vi "SRV_Update Main Window Title and Open Window.vi"(0 "VI ref":refnum<vi>, 11 "error in (no error)":errorcluster, 12 "FP.Open? (T)":bool=TRUE) -> (4 "VI ref out":refnum<vi>, 15 "error out":errorcluster)   [LabVIEW 2009]
doc: "Updates the FrontPanel.Title property of the referenced VI. The title will be \"SRV Main Controller\" plus a version number if one exists at the end of the VI filename.\n\n\nAuthor: Mike Schultz - Logic PD"
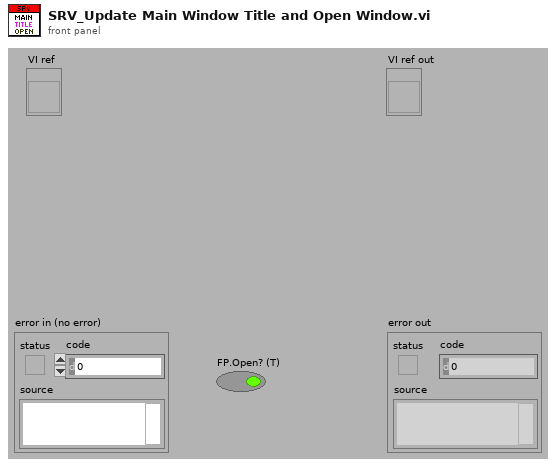
[diagram p1: front panel]
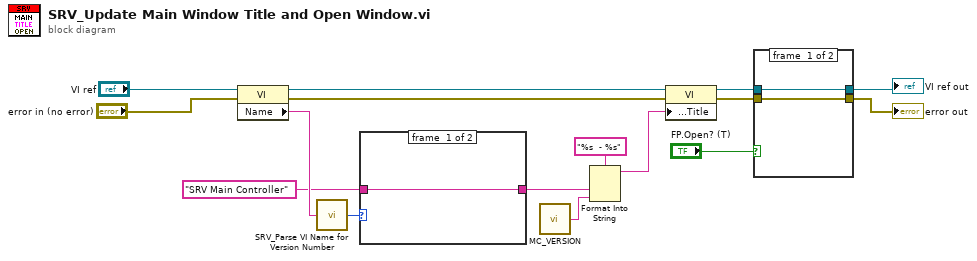
[diagram p0: block diagram]
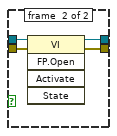
[diagram p2: hidden frame]
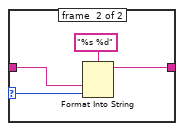
[diagram p3: hidden frame]
diagram:
  n1 = property class="VI"(reference="VI ref", error in="error in (no error)") -> (reference out=w12:refnum<vi>, error out=w11:errorcluster, "Name"=w15:string)
  n2 = call "SRV_Parse VI Name for Version Number.vi"("VI Name"=w15) -> ("Version Number"=w14:i32)  [unwired: 14 in]
  n3 = case shown="Default" w14 {
    selector: w14 -> [_ w18]
    tunnel: "SRV Main Controller" -> [w17 w20]
    tunnel: [w17 w19] -> w4
    frame #0 {
    }
    frame #1 {
      n4 = Format Into String(format string="%s %d", w20, w18) -> (resulting string=w19:string)  [unwired: 2 in, 1 out]
    }
  }
  n5 = call "MC_VERSION.vi"() -> ("MC Version"=w2:string)
  n6 = Format Into String(format string="%s  - %s", w4, w2) -> (resulting string=w3:string)  [unwired: 2 in, 1 out]
  n7 = property class="VI"(reference=w12, error in=w11, "Front Panel.Title"=w3) -> (reference out=w7:refnum<vi>, error out=w9:errorcluster)
  n8 = case shown="True" "FP.Open? (T)" {
    tunnel: w9 -> [w23 w27]
    tunnel: [w23 w26] -> w8
    tunnel: w7 -> [w22 w25]
    tunnel: [w22 w24] -> w6
    frame #0 {
    }
    frame #1 {
      n9 = invoke class="VI" method="FP.Open"(reference=w25, error in=w27) -> (reference out=w24:refnum<vi>, error out=w26:errorcluster)  [unwired: 3 in, 3 out]
    }
  }
  "error out" <- w8
  "VI ref out" <- w6
